vi "FrameParseSeparateHeader.vi"(0 "DataBuffer":string) -> (14 "FoundHeader":bool)   [LabVIEW 2017, in "STOMP.lvclass"]
uses:
  STOMP.lvclass
  <vilib>/regexp/Match Regular Expression.xnode
panel:
  in  "error in":errorcluster
  out "error out":errorcluster
  out "RemainingData":string
  out "Headers":string
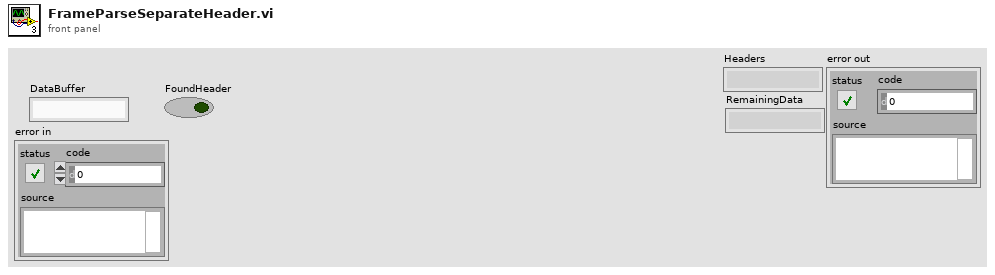
[diagram p1: front panel]
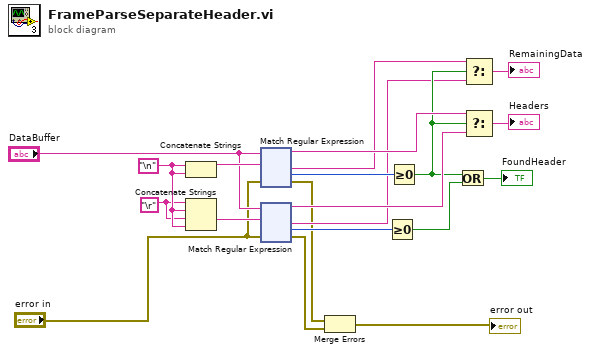
[diagram p0: block diagram]
diagram:
  w13 = "\n"
  w12 = "\r"
  n1 = Concatenate Strings(w13, w13) -> (w15:string)
  n2 = Concatenate Strings(w12, w13, w12, w13) -> (w16:string)
  n3 = xnode "Match Regular Expression"("input string"="DataBuffer", "regular expression"=w15, "error in"="error in") -> ("before match"=w10:string, "after match"=w7:string, "offset past match"=w17:i32, "error out"=w2:errorcluster)  [unwired: 3 in, 1 out]
  n4 = xnode "Match Regular Expression"("input string"="DataBuffer", "regular expression"=w16, "error in"="error in") -> ("before match"=w11:string, "after match"=w6:string, "offset past match"=w18:i32, "error out"=w4:errorcluster)  [unwired: 3 in, 1 out]
  n5 = Merge Errors(w2, w4) -> (→"error out":errorcluster)
  n6 = Greater Or Equal To 0?(x=w18) -> (x >= 0?=w19:bool)
  n7 = Greater Or Equal To 0?(x=w17) -> (x >= 0?=w8:bool)
  n8 = Or(x=w8, y=w19) -> (x .or. y?=→"FoundHeader":bool)
  n9 = Select(t=w7, s=w8, f=w6) -> (s? t:f=→"RemainingData":string)
  n10 = Select(t=w10, s=w8, f=w11) -> (s? t:f=→"Headers":string)
